vi "Camera Steer.vi"(1 "Reinit?":bool, 2 "Target X":dbl) -> (0 "Steer Amount":dbl)   [LabVIEW 2013]
uses:
  <vilib>/addons/control/pid/NI_PID_pid.lvlib
  <vilib>/addons/control/pid/pid.llb/PID (DBL).vi
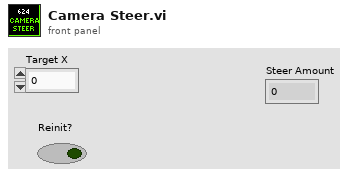
[diagram p1: front panel]
types:
  T1 = cluster{"proportional gain (Kc)":dbl, "integral time (Ti, min)":dbl, "derivative time (Td, min)":dbl}
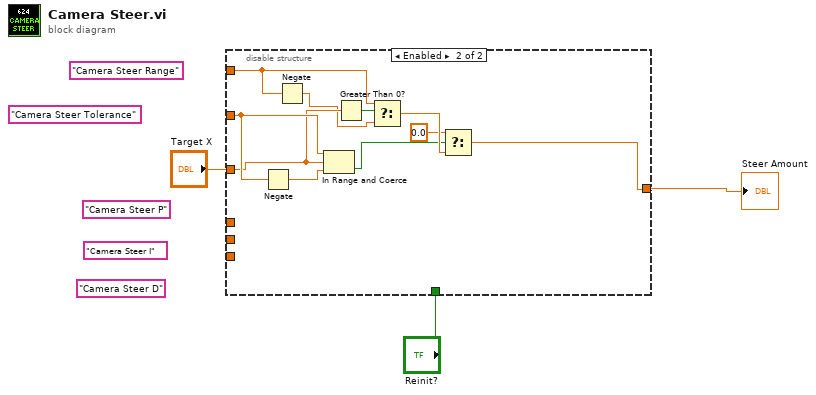
[diagram p0: block diagram]
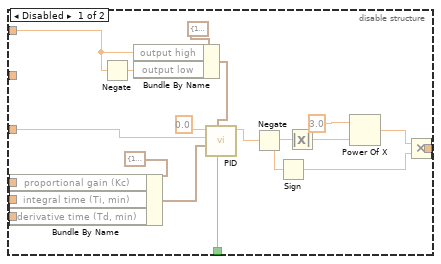
[diagram p2: hidden frame]
diagram:
  w2 = "Camera Steer Tolerance" ("Name")
  w4 = "Camera Steer D" ("Name")
  w5 = "Camera Steer I" ("Name")
  w6 = "Camera Steer P" ("Name")
  w7 = "Camera Steer Range" ("Name")
  n1 = disable-structure shown="Enabled" {
    disable-tunnel: "Reinit?" -> [w28 _]
    disable-tunnel: "Target X" -> [w27 w36]
    disable-tunnel: _ -> [w23 w34]
    disable-tunnel: _ -> [w19 _]
    disable-tunnel: _ -> [w18 _]
    disable-tunnel: _ -> [w17 _]
    disable-tunnel: [w11 w29] -> w3
    disable-tunnel: [_ w37] -> w1
    frame Disabled {
      n2 = Bundle By Name(cluster=T1 {"proportional gain (Kc)"=1.0, "integral time (Ti, min)"=0.01, "derivative time (Td, min)"=0.0} ("PID gains"), "proportional gain (Kc)"=w17, "integral time (Ti, min)"=w19, "derivative time (Td, min)"=w18) -> (w20:T1)
      n3 = Negate(x=w23) -> (-x=w22:dbl)
      n4 = Bundle By Name(cluster=cluster{"output high":dbl, "output low":dbl} {"output high"=100.0, "output low"=-100.0} ("output range"), "output high"=w23, "output low"=w22) -> (w24:cluster{"output high":dbl, "output low":dbl})
      n5 = call-poly <vilib>:"PID.vi"("reinitialize? (F)"=w28, "output range"=w24, "PID gains"=w20, "process variable"=w27, "setpoint"=0.0) -> ("output"=w16:dbl)  [unwired: 5 in, 1 out]
      n6 = Negate(x=w16) -> (-x=w10:dbl)
      n7 = Sign(1:w10) -> (0:w12:dbl)
      n8 = Absolute Value(x=w10) -> (abs(x)=w14:dbl)
      n9 = Power Of X(1:w14, 2:3.0 ("y")) -> (0:w13:dbl)
      n10 = Multiply(x=w13, y=w12) -> (x*y=w11:dbl)
    }
    frame Enabled {
      n11 = Negate(x=w37) -> (-x=w38:dbl)
      n12 = Negate(x=w34) -> (-x=w33:dbl)
      n13 = In Range and Coerce(upper limit=w37, x=w36, lower limit=w38) -> (In Range?=w31:bool)  [unwired: 1 out]
      n14 = Greater Than 0?(x=w36) -> (x > 0?=w35:bool)
      n15 = Select(t=w34, s=w35, f=w33) -> (s? t:f=w32:dbl)
      n16 = Select(t=0.0, s=w31, f=w32) -> (s? t:f=w29:dbl)
    }
  }
  "Steer Amount" <- w3
